vi "Pos ctrl window globals.vi"() -> ()   [LabVIEW 2020]
uses:
  Typedefs/Pos Ctrl window refs cluster.ctl
  <userlib>/My Palettes.lib/Custom Controls/Directional Arrow Buttons/Arrow button-North.ctl
  Typedefs/Axis of movement.ctl
  Typedefs/Movement mode.ctl
panel:
  in  "Movement mode":T1=enum."Move the feature"
  in  "Axis of movement":T2=enum."X-axis"
  out "Window is open":bool
  out "Bring to front":bool
  in  "Minimum allowed speed":i32=1
  in  "Maximum allowed speed":i32=100
  in  "Speed setting increment":i32=1
  in  "+- Z Limit (um)":sgl=150.0 min=0.1 step=0.1
  in  "Z step (um)":sgl=0.1 min=0.1
  in  "Step = size of image":bool
  in  "XY step (um)":sgl=0.1 min=0.1
  in  "Dequeue timeout (sec)":dbl=8.0
  in  "Pos ctrl window refs":T3
  # "#PositionCtrl - Save/Load these global variable values from file."
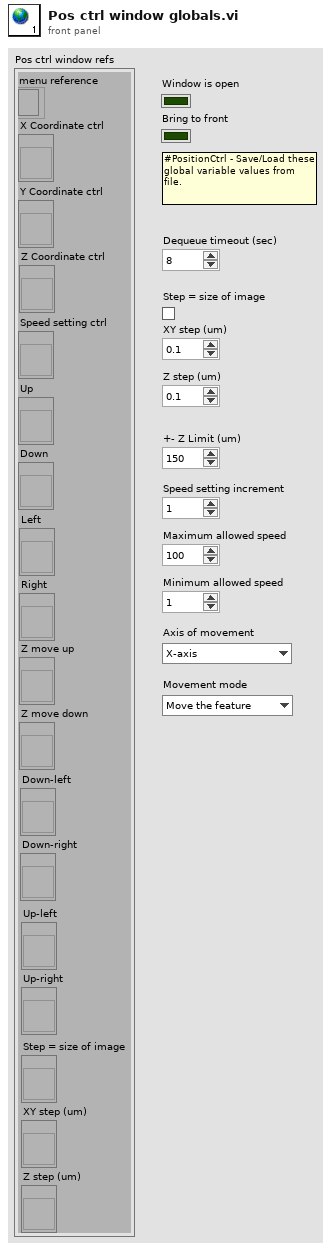
[diagram p1: front panel]
types:
  T1 = typedef "Movement mode.ctl" = enum16{"Move the frame", "Move the feature"}
  T2 = typedef "Axis of movement.ctl" = enum16{"None", "X-axis", "Y-Axis", "-45 deg Axis", "+45 deg Axis", "Z-Axis"}
  T3 = typedef "Pos Ctrl window refs cluster.ctl" = cluster{"menu reference":refnum<k9>, "X Coordinate ctrl":refnum<vi>, "Y Coordinate ctrl":refnum<vi>, "Z Coordinate ctrl":refnum<vi>, "Speed setting ctrl":refnum<vi>, "Up":refnum<vi>, "Down":refnum<vi>, "Left":refnum<vi>, "Right":refnum<vi>, "Z move up":refnum<vi>, "Z move down":refnum<vi>, "Down-left":refnum<vi>, "Down-right":refnum<vi>, "Up-left":refnum<vi>, "Up-right":refnum<vi>, "Step = size of image":refnum<vi>, "XY step (um)":refnum<vi>, "Z step (um)":refnum<vi>}
diagram:
